vi "CreateHTML.vi"(0 "reference in":refnum<class "Progressbar.lvclass">, 2 "VI Name":string, 5 "error in (no error)":errorcluster) -> (13 "script dependencies":string[](array[string]), 14 "reference out":refnum<class "Progressbar.lvclass">, 15 "HTML":string, 16 "js variables":string, 17 "js code for controls":string, 18 "js code for indicators":string, 19 "error out":errorcluster)   [LabVIEW 2014, in "Progressbar.lvclass"]
uses:
  Progressbar.lvclass
  Object_class/Object.lvclass
  Control_class/Control.lvclass
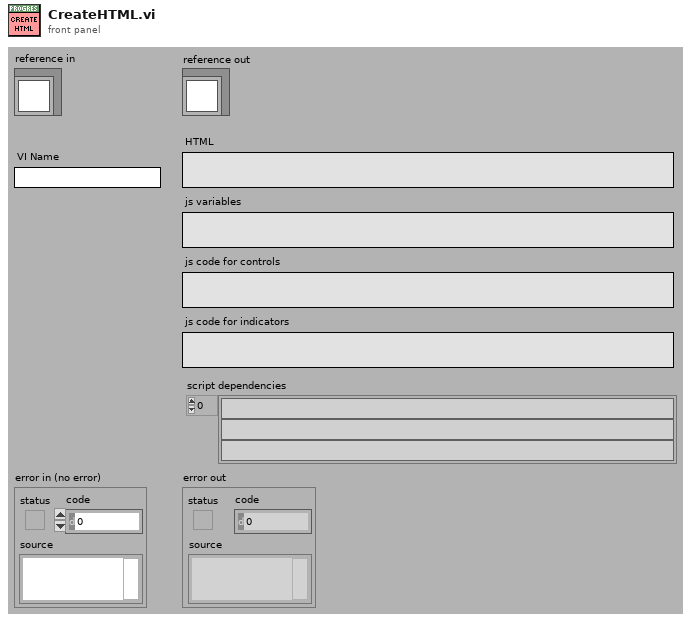
[diagram p1: front panel]
types:
  T1 = typedef "Object.lvclass/Attributes.ctl" = cluster{"UID":i32, "Type":string, "Coordinates":T2, "Reference":refnum<vi>}
  T2 = typedef "Object.lvclass/Coordinates.ctl" = cluster{"Left":i32, "Top":i32, "Height":u32, "Width":u32}
  T3 = typedef "Control.lvclass/Attributes.ctl" = cluster{"Description":string, "Indicator":bool, "Default Value":variant, "Control Index":i32, "Label":refnum<class "Text.lvclass">, "Caption":refnum<class "Text.lvclass">, "Use Picture":bool, "Image1 b64":string, "Image2 b64":string}
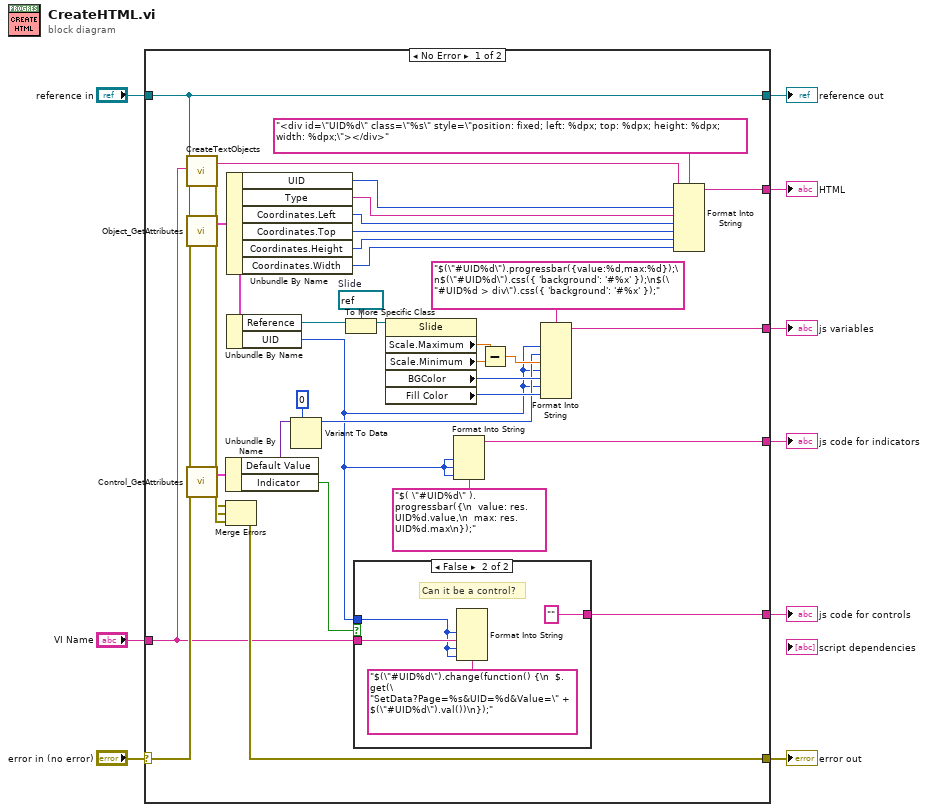
[diagram p0: block diagram]
diagram:
  n1 = case shown="No Error" "error in (no error)" {
    selector: "error in (no error)" -> [w45 w51]
    tunnel: [w41 w51] -> w8
    tunnel: [w28 w50] -> w6
    tunnel: "reference in" -> [w28 w50]
    tunnel: [w35 _] -> w5
    tunnel: [w30 _] -> w4
    tunnel: [w32 _] -> w3
    tunnel: "VI Name" -> [w27 _]
    tunnel: [w17 _] -> w1
    frame No Error {
      w22 = refnum<vi> refnum  # Slide
      n2 = call-dynamic "CreateTextObjects.vi"("reference in"=w28, "VI Name"=w27) -> ("HTML"=w29:string, "error out"=w42:errorcluster)  [unwired: 15 in, 1 out]
      n3 = call "Object_GetAttributes.vi"("reference in"=w28, "error in (no error)"=w45) -> ("Data"=w19:T1, "error out"=w43:errorcluster)  [unwired: 14 in, 2 out]
      n4 = call "Control_GetAttributes.vi"("reference in"=w28, "error in (no error)"=w45) -> ("Data"=w34:T3, "error out"=w44:errorcluster)  [unwired: 14 in, 2 out]
      n5 = Unbundle By Name(w34) -> ("Default Value"=w26:variant, "Indicator"=w33:bool)
      n6 = Merge Errors(w42, w43, w44) -> (w41:errorcluster)
      n7 = Unbundle By Name(w19) -> ("UID"=w39:i32, "Type"=w38:string, "Coordinates.Left"=w37:i32, "Coordinates.Top"=w36:i32, "Coordinates.Height"=w24:u32, "Coordinates.Width"=w23:u32)
      n8 = Unbundle By Name(w19) -> ("Reference"=w18:refnum<vi>, "UID"=w12:i32)
      n9 = Variant To Data(type=0, Variant=w26) -> (data=w13:i32)  [unwired: 1 in, 1 out]
      n10 = To More Specific Class(target class=w22, reference=w18) -> (specific class reference=w21:refnum<vi>)  [unwired: 1 in, 1 out]
      n11 = case shown="False" w33 {
        tunnel: w12 -> [_ w47]
        tunnel: w27 -> [_ w49]
        tunnel: [_ ""] -> w32
        frame True {
        }
        frame False {
          # "Can it be a control?"
          n12 = Format Into String(format string="$(\"#UID%d\").change(function() {\n  $.get(\"SetData?Page=%s&UID=%d&Value=\" + $(\"#UID%d\").val())\n});", w47, w49, w47, w47) -> ()  [unwired: 2 in, 2 out]
        }
      }
      n13 = property class="Slide"(reference=w21) -> ("Scale.Maximum"=w11:dbl, "Scale.Minimum"=w10:dbl, "BGColor"=w16:u32, "Fill Color"=w15:u32)  [unwired: 1 in, 2 out]
      n14 = Format Into String(format string="$( \"#UID%d\" ).progressbar({\n  value: res.UID%d.value,\n  max: res.UID%d.max\n});", w12, w12, w12) -> (resulting string=w30:string)  [unwired: 2 in, 1 out]
      n15 = Subtract(x=w11, y=w10) -> (x-y=w14:dbl)
      n16 = Format Into String(format string="$(\"#UID%d\").progressbar({value:%d,max:%d});\n$(\"#UID%d\").css({ 'background': '#%x' });\n$(\"#UID%d > div\").css({ 'background': '#%x' });", w12, w13, w14, w12, w16, w12, w15) -> (resulting string=w17:string)  [unwired: 2 in, 1 out]
      n17 = Format Into String(format string="<div id=\"UID%d\" class=\"%s\" style=\"position: fixed; left: %dpx; top: %dpx; height: %dpx; width: %dpx;\"></div>", initial string=w29, w39, w38, w37, w36, w24, w23) -> (resulting string=w35:string)  [unwired: 1 in, 1 out]
    }
    frame Error {
    }
  }
  "error out" <- w8
  "reference out" <- w6
  "HTML" <- w5
  "js variables" <- w1
  "js code for controls" <- w3
  "js code for indicators" <- w4
